vi "MAIN Z Test.vi"() -> ()   [LabVIEW 2017]
uses:
  C:/Program Files (x86)/National Instruments/LabVIEW 2017/examples/Instrument IO/Serial/support/Serial - Settings.ctl
  <vilib>/Instr/_visa.llb/VISA Configure Serial Port (Instr).vi
panel:
  in  "Z_M_Center":bool
  in  "Z_M_Fokus":bool
  in  "Z_M_Position":bool
  in  "Z_D_absWinkel":bool
  in  "Z_M_Trigger":bool
  in  "Stopp":bool
  in  "Pos (0 - 72000)":i32
  in  "Winkel (gon)":i32 min=0 max=15000
  out "Antwort":string
  in  "VISA-Ressourcenname":refnum<visa-resource-name>="COM13"
  in  "Einstellungen des seriellen Ports":T1={"Baudrate"=19200, "Datenbits"=8, "Parität"=enum."None", "Stoppbits"=10, "Ablaufsteuerung"=0} {"Ablaufsteuerung" items=["Keine"=0, "XON/XOFF"=1, "RTS/CTS"=2, "DTR/DSR"=4]; "Stoppbits" items=["1,0"=10, "1,5"=15, "2,0"=20]; "Datenbits" min=5 max=8 step=1; "Baudrate" items=["75"=75, "110"=110, "134"=134, "150"=150, "300"=300, "600"=600, "1200"=1200, "1800"=1800, "2400"=2400, "4800"=4800, "7200"=7200, "9600"=9600, "14400"=14400, "19200"=19200, "28800"=28800, "38400"=38400, "56000"=56000, "57600"=57600, "115200"=115200, "128000"=128000, "230400"=230400]}
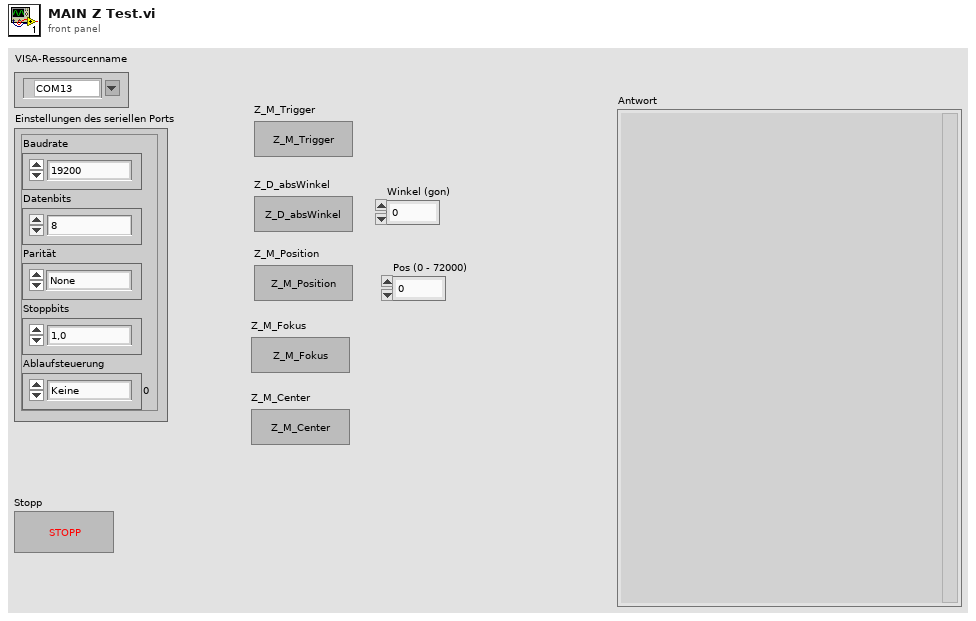
[diagram p1: front panel]
types:
  T1 = typedef "Serial - Settings.ctl" = cluster{"Baudrate":u32, "Datenbits":u16, "Parität":enum16{"None", "Odd", "Even", "Mark", "Space"}, "Stoppbits":u16, "Ablaufsteuerung":u16}
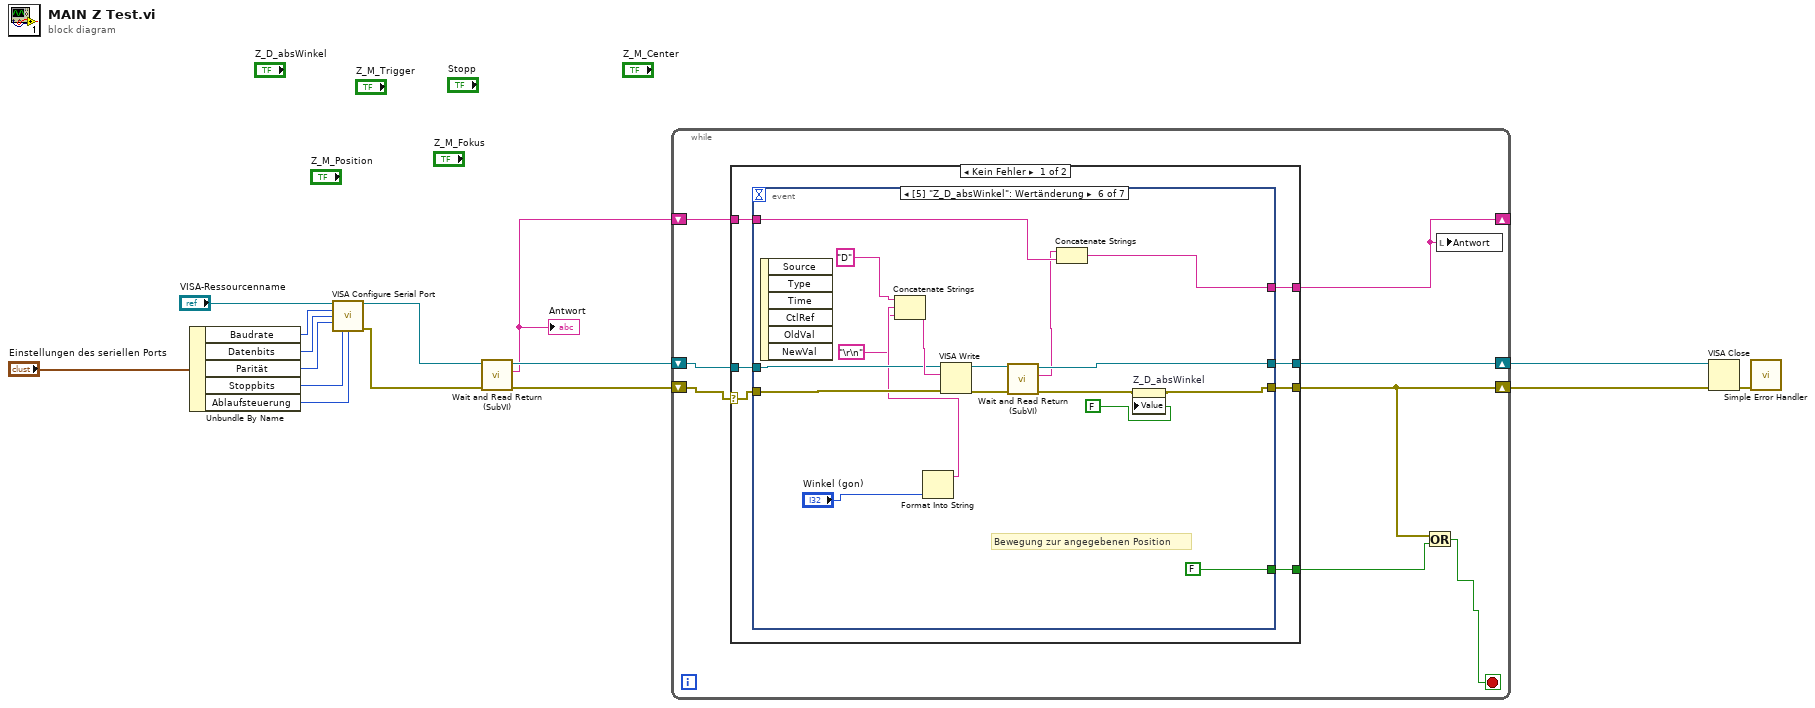
[diagram p0: block diagram]
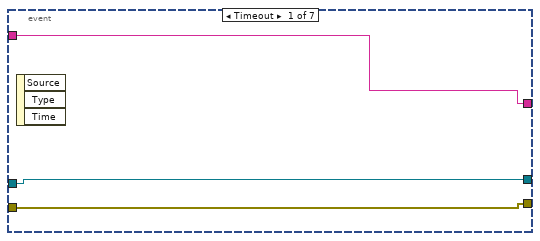
[diagram p2: hidden frame]
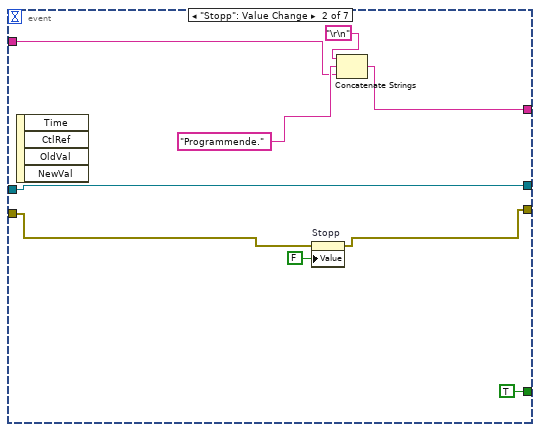
[diagram p3: hidden frame]
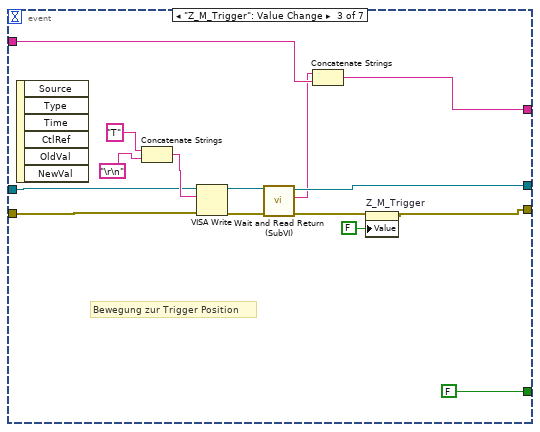
[diagram p4: hidden frame]
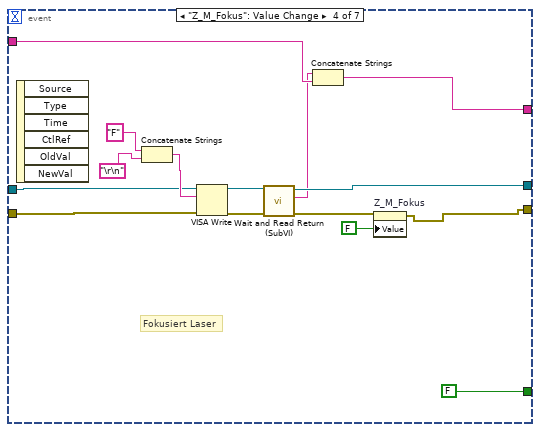
[diagram p5: hidden frame]
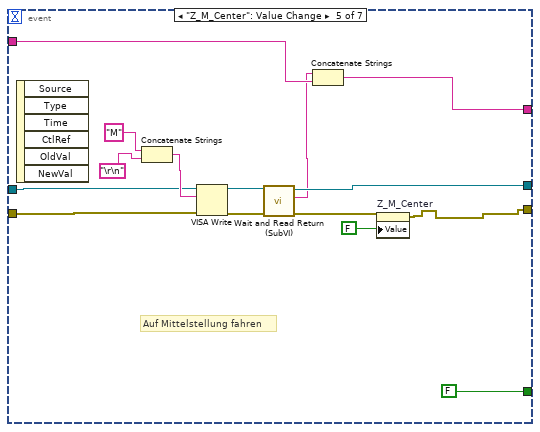
[diagram p6: hidden frame]
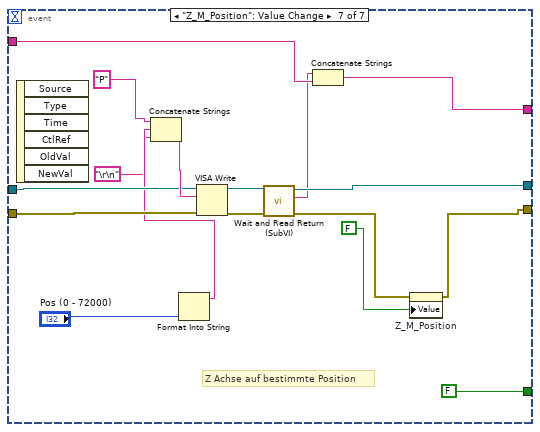
[diagram p7: hidden frame]
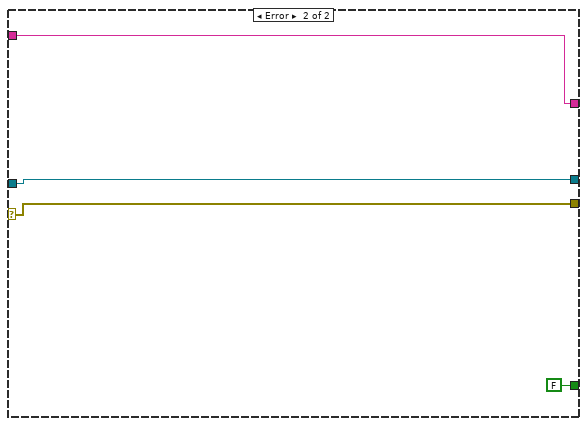
[diagram p8: hidden frame]
diagram:
  n1 = Unbundle By Name("Einstellungen des seriellen Ports") -> ("Baudrate"=w10:u32, "Datenbits"=w11:u16, "Parität"=w12:enum16{"None", "Odd", "Even", "Mark", "Space"}, "Stoppbits"=w13:u16, "Ablaufsteuerung"=w8:u16)
  n2 = call-poly "VISA Configure Serial Port"("VISA resource name"="VISA-Ressourcenname", "baud rate (9600)"=w10, "data bits (8)"=w11, "parity (0:none)"=w12, "stop bits (10: 1 bit)"=w13, "flow control (0:none)"=w8) -> ("VISA resource name out"=w7:refnum<visa-resource-name>, "error out"=w6:errorcluster)  [unwired: 4 in, 4 out]
  n3 = call "Wait and Read Return (SubVI).vi"("Fehler (Eingang, kein Fehler)"=w6, "VISA-Referenz (Eingang)"=w7) -> ("Fehler (Ausgang)"=w4:errorcluster, "Antwort"=w1:string, "VISA-Referenz (Ausgang)"=w5:refnum<visa-resource-name>)  [unwired: 7 in]
  "Antwort" <- w1
  n4 = while {
    shift-right: [w22] -> w3
    shift-left: w5 -> [w23]
    shift-right: [w19] -> w2
    shift-left: w4 -> [w16]
    shift-right: [w20] -> _
    shift-left: w1 -> [w21]
    stop <- w17 stop-if-true
    n5 = case shown="Kein Fehler" w16 {
      selector: w16 -> [w24 w125]
      tunnel: w23 -> [w30 w124]
      tunnel: [w29 w124] -> w22
      tunnel: w21 -> [w28 w123]
      tunnel: [w27 w123] -> w20
      tunnel: [w26 w125] -> w19
      tunnel: [w25 FALSE] -> w18
      frame No Error {
        n6 = event shown="[5] \"Z_D_absWinkel\": Wertänderung" {
          selector: _ -> [_ _ _ _ _ _ _]
          dyn-events: _ -> [_ _ _ _ _ _ _]
          timeout: _ -> [_ _ _ _ _ _ _]
          tunnel: w30 -> [w33 w42 w52 w67 w82 w101 w118]
          tunnel: w24 -> [w32 w39 w51 w66 w81 w100 w117]
          tunnel: [w33 w42 w50 w65 w80 w99 w116] -> w29
          tunnel: [w32 w38 w45 w60 w75 w93 w109] -> w26
          tunnel: [w31 w40 w48 w63 w78 w97 w114] -> w27
          tunnel: [_ TRUE FALSE FALSE FALSE FALSE FALSE] -> w25
          tunnel: w28 -> [w31 w35 w44 w59 w74 w90 w107]
          event Timeout {
            n7 = event-data() -> ()  [unwired: 1 in, 3 out]
          }
          event "Stopp": Value Change {
            n8 = event-data() -> ()  [unwired: 1 in, 4 out]
            n9 = property on="Stopp" class="Bool. (strikt)"(error in=w39, "Value"=FALSE ("Stopp")) -> (error out=w38:errorcluster)  [unwired: 1 in, 1 out]
            n10 = Concatenate Strings("\r\n", "Programmende." ("String"), w35) -> (w40:string)
          }
          event "Z_M_Trigger": Value Change {
            # "Bewegung zur Trigger Position"
            n11 = event-data() -> ()  [unwired: 1 in, 6 out]
            n12 = Concatenate Strings("T" ("Schreibpuffer"), "\r\n") -> (w55:string)
            n13 = VISA Write(VISA resource name=w52, write buffer=w55, error in (no error)=w51) -> (VISA resource name out=w54:refnum<visa-resource-name>, error out=w53:errorcluster)  [unwired: 1 out]
            n14 = call "Wait and Read Return (SubVI).vi"("Fehler (Eingang, kein Fehler)"=w53, "VISA-Referenz (Eingang)"=w54) -> ("Fehler (Ausgang)"=w46:errorcluster, "Antwort"=w43:string, "VISA-Referenz (Ausgang)"=w50:refnum<visa-resource-name>)  [unwired: 7 in]
            n15 = Concatenate Strings(w43, w44) -> (w48:string)
            n16 = property on="Z_M_Trigger" class="Bool. (strikt)"(error in=w46, "Value"=FALSE ("XY_M_Trigger")) -> (error out=w45:errorcluster)  [unwired: 1 in, 1 out]
          }
          event "Z_M_Fokus": Value Change {
            # "Fokusiert Laser"
            n17 = event-data() -> ()  [unwired: 1 in, 6 out]
            n18 = Concatenate Strings("F" ("Schreibpuffer"), "\r\n") -> (w70:string)
            n19 = VISA Write(VISA resource name=w67, write buffer=w70, error in (no error)=w66) -> (VISA resource name out=w69:refnum<visa-resource-name>, error out=w68:errorcluster)  [unwired: 1 out]
            n20 = call "Wait and Read Return (SubVI).vi"("Fehler (Eingang, kein Fehler)"=w68, "VISA-Referenz (Eingang)"=w69) -> ("Fehler (Ausgang)"=w61:errorcluster, "Antwort"=w58:string, "VISA-Referenz (Ausgang)"=w65:refnum<visa-resource-name>)  [unwired: 7 in]
            n21 = Concatenate Strings(w58, w59) -> (w63:string)
            n22 = property on="Z_M_Fokus" class="Bool. (strikt)"(error in=w61, "Value"=FALSE ("XY_M_Trigger")) -> (error out=w60:errorcluster)  [unwired: 1 in, 1 out]
          }
          event "Z_M_Center": Value Change {
            # "Auf Mittelstellung fahren"
            n23 = event-data() -> ()  [unwired: 1 in, 6 out]
            n24 = Concatenate Strings("M" ("Schreibpuffer"), "\r\n") -> (w85:string)
            n25 = VISA Write(VISA resource name=w82, write buffer=w85, error in (no error)=w81) -> (VISA resource name out=w84:refnum<visa-resource-name>, error out=w83:errorcluster)  [unwired: 1 out]
            n26 = call "Wait and Read Return (SubVI).vi"("Fehler (Eingang, kein Fehler)"=w83, "VISA-Referenz (Eingang)"=w84) -> ("Fehler (Ausgang)"=w76:errorcluster, "Antwort"=w73:string, "VISA-Referenz (Ausgang)"=w80:refnum<visa-resource-name>)  [unwired: 7 in]
            n27 = Concatenate Strings(w73, w74) -> (w78:string)
            n28 = property on="Z_M_Center" class="Bool. (strikt)"(error in=w76, "Value"=FALSE ("XY_M_Trigger")) -> (error out=w75:errorcluster)  [unwired: 1 in, 1 out]
          }
          event "Z_D_absWinkel": Value Change {
            # "Bewegung zur angegebenen Position"
            n29 = event-data() -> ()  [unwired: 1 in, 6 out]
            n30 = Format Into String("Winkel (gon)") -> (resulting string=w94:string)  [unwired: 3 in, 1 out]
            n31 = Concatenate Strings("D" ("Schreibpuffer"), w94, "\r\n") -> (w104:string)
            n32 = VISA Write(VISA resource name=w101, write buffer=w104, error in (no error)=w100) -> (VISA resource name out=w103:refnum<visa-resource-name>, error out=w102:errorcluster)  [unwired: 1 out]
            n33 = call "Wait and Read Return (SubVI).vi"("Fehler (Eingang, kein Fehler)"=w102, "VISA-Referenz (Eingang)"=w103) -> ("Fehler (Ausgang)"=w92:errorcluster, "Antwort"=w89:string, "VISA-Referenz (Ausgang)"=w99:refnum<visa-resource-name>)  [unwired: 7 in]
            n34 = Concatenate Strings(w89, w90) -> (w97:string)
            n35 = property on="Z_D_absWinkel" class="Bool. (strikt)"(error in=w92, "Value"=FALSE ("XY_M_Trigger")) -> (error out=w93:errorcluster)  [unwired: 1 in, 1 out]
          }
          event "Z_M_Position": Value Change {
            # "Z Achse auf bestimmte Position"
            n36 = event-data() -> ()  [unwired: 1 in, 6 out]
            n37 = Format Into String("Pos (0 - 72000)") -> (resulting string=w112:string)  [unwired: 3 in, 1 out]
            n38 = Concatenate Strings("P" ("Schreibpuffer"), w112, "\r\n") -> (w121:string)
            n39 = VISA Write(VISA resource name=w118, write buffer=w121, error in (no error)=w117) -> (VISA resource name out=w120:refnum<visa-resource-name>, error out=w119:errorcluster)  [unwired: 1 out]
            n40 = call "Wait and Read Return (SubVI).vi"("Fehler (Eingang, kein Fehler)"=w119, "VISA-Referenz (Eingang)"=w120) -> ("Fehler (Ausgang)"=w110:errorcluster, "Antwort"=w106:string, "VISA-Referenz (Ausgang)"=w116:refnum<visa-resource-name>)  [unwired: 7 in]
            n41 = Concatenate Strings(w106, w107) -> (w114:string)
            n42 = property on="Z_M_Position" class="Bool. (strikt)"(error in=w110, "Value"=FALSE ("XY_M_Trigger")) -> (error out=w109:errorcluster)  [unwired: 1 in, 1 out]
          }
        }
      }
      frame Error {
      }
    }
    n43 = Or(x=w19, y=w18) -> (x .or. y?=w17:bool)
    n44 = local write "Antwort"(w20) -> ()
  }
  n45 = VISA Close(VISA resource name=w3, error in (no error)=w2) -> (error out=w15:errorcluster)
  n46 = call <vilib>:"Simple Error Handler.vi"("error in (no error)"=w15) -> ()  [unwired: 4 in, 5 out]
